vi "micUnbundle.vi"   [LabVIEW 2011]
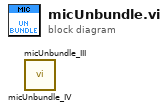
[diagram p0: block diagram]
diagram:
  n1 = call "micUnbundle_IV.vi"() -> ()  [unwired: 11 in, 5 out]
  n2 = call "micUnbundle_III.vi"() -> ()  [unwired: 12 in, 4 out]
